vi "Day 3-1.vi"() -> ()   [LabVIEW 2022 SP3]
uses:
  <vilib>/Utility/miscctls.llb/LVMapReplaceAction.ctl
panel:
  out "sum 2":i32
  out "sum":i32
  in  "String":string="..172..............................454..46.......507..........809......923.778..................793..............137.............238........\n............*.........712........=.......*................515.*...........*.......690.........../..........658.........=.........*..........\n.........823.835........%.........710.....749........134..%............................#812...&.....925.../..........276.......386..........\n519..................13......341.................481....=.....$............-.......211.......92.......*.....................................\n............832*105..@........$..................*.........797.....535..932.........*....152...........123.........678.540...........-...6..\n....&..948..........................271....-....228..79.26.........................733...=...715............27.586........*.......883...*...\n..172.......=..+.............88&....%....340.55.....+.............465..398......=..................585.......*....*812...347................\n...........374.462.......166..................*...........786........*....*910..675.................*.....149................653*....+80....\n.......*............680.....*......876.........864..................259.................124.169....799............608..*.........98......951\n....615.......*....%.....151.........*....#802........$.......680......................../...............857........-.901...............*...\n..............3.................637..493...........926....636..*.....350........881.........699......886.../.458...........#..474*409...246.\n...&...336......922............*..........370..............$..581....*.....335.*.......608$..*..11.......$....-..........928................\n...50..*.........*...........978...453.....*.......-..22..........298.......*...711.........794...*...267............44*.......460....*.....\n...................................*........534..797....-.............61....272.....@874..........892.....707.............230....*..72.537..\n....................405............309..........................221./..*....................872%.......75..*......237.....*.................\n..208.176..239.........*172.............795.............670.......*..9..504......*.717..641........908*....975.....*......130...............\n.....*....*.......711$....................*..54.....494..../.333.882...........282....@.......927*....../.......555..983*...........479.....\n.915......670.524................866...862..@.........*../....*...................................72.901..................995..........&....\n...*..%.......*.....71.............*..................33.350.796.....612.............#..463..............*399.....=.......*......309........\n....8..951.886......@......41*......606.680...787................605*.....892.......219.*........972..846.........377....644................\n..............................718........*.......*.......355*688............*.145...................*.......576.............................\n..........867.*.....................+...974...148..........................87.#........500&...534..986..269...*.....576....302....+.........\n........@......504.......-........652.........................104....@502......................*...............691.*.........*.423..706..402\n.286..218.882........-....579......................320.....=...-..........48.393.....202......758.....242..951..............................\n....*.....*.....$..943.............928.....*......*......310......&........*....*...*......=..............*......295*133....................\n..698...331...859.......91.........#....815....822..............39..........833....749...591...........455....*..........&30....*...........\n............*............+..............................117............................%........727........256.439...19.......478...........\n......67.595...599.........442...997..187.................@.596..276..141.597*792...780.........*......*.............@..............#.......\n266@.............-..713.....*....*.......=..783...564*.......*.......@.........................839......255.............636......749..%.....\n........+............*.....963.926.39../......&.......274...228..../.....812.........487@.24.............................*..*..........348..\n...618...364.936.....708...........*....63..&.......................212....-..191..............798................*....591..906.............\n......./.....@...............591...127.......491...141..*.....+...............*......339.@483........204*......871.465..................%...\n....890..................997*............723........$..675..465..............372.875*.........%..........534.............209.......*.....648\n..............+................139*..........273..................../7.....-..............854.920...968%..........384......%.......830......\n......+632...273.......132*........793.........................207..........952..../..66..*........................#...........@............\n.......................................162..................35.*.................22..*....234..........468...................#.750..........\n.....15...161.....................93....@...818..-580........*.449...................125...........129....*................723......365.....\n.....-....*.......678.........&21...=....../..............547.......$.........701....................#.....845.........................#....\n743........634...*.................................................679...........*176......979....................928.......$..848..........\n...............107....296....845.....*..........@...........................69..............$..442.........960/...........311.*.............\n.........................*............519.....58..............248.......582*........403.......*........929..............-......486.......151\n....-390....396.........279.......718............449.....794..#..............+......*......251...980....../.../...328..476..................\n.............*.....................-......../...*...........*...292.........188...&..112............*315.....529............................\n713..........860......114.743&.......368.776...195.........850.=................943............543...................483*625................\n......889........=.../.................*.............916.............201............-...............426&....627..............284............\n.452...........579...........786.961.15.......488.......*373.....830*......947.645.189........367.................$..../551.................\n....*.....99*........388.793...*...*....578..../...........................*...%.......-497.........@221..720...885.........588....692......\n....................*........903..81.......*.......*........=./....615.....202...355........997-..........*................$.........*......\n...........780.@....259.439.................483....596...490..415....*............-........................683........*371...&644..964......\n.......796......161.......*..#884....................................458.247.500........145.895.62.742.267..........16......................\n......+............../.998...........173..511............552*847...%.....&.........+651..*.....*........*.....108........+..............*975\n.444.....560.297...149..............*....*......*...................173...................365............986.$............271...182...26....\n....*84....*......................#..471.696.736.107....974...-614............................../...%930..........................+......364\n............800...-155..235......446...................*....................286.......822../...199............670-....................%.....\n....882.................*.................521....*20.282.............641.......*..703*.....887......513*271....................+819..100....\n.99..*........933*...649.......407............922...............-......*....681.............................*....#426...204.................\n.....112................../.....*...819.94......................689...652...........182.933.858.............711...............610.....*437..\n.540..........#.........740...500....*...$....184.......................................*....#.......386...........................668......\n....$..........719..695...........824............&...882...........@......811........771.........142*.........867.667.*299.....143..........\n425....120.............*....401........................*....75..2..551.....*...719....................44..141...+..............+............\n...%..*..........963....209..&.....913.................871..=............%.904.........365.244.495....*....*........19......................\n.....971.........=.............883*.........225.967.............#......44.................*.....*..182......830.....@..190............487...\n...................................../........*.%........93....577..%......541.....*456.....370.52......................%.............@.....\n..82......396....................927..887...268...........&..........517...................%...............753................+.............\n.........*..........................*.........................................607..493.479.........521......*.....680*58..&....879..........\n......951.................136.&....585.........69....933.........25......265......*............923...&......5.............624........109....\n...........826..............$..407..............*...............*...+...........772.=...........*.............................628...........\n.......293..*...420...................................140.......728..815.196.-.......470.....403.................807..........*...99.....443\n......-.....732...*.........795....35........18.........*................*....789................931................-.52....727....*....*...\n.................477..@682..*.......*...118.........539.................844......................*...481.....%..........*..........863...773\n...479&......................585..817...@...........*...16*244...826*..........427...............694.......834.......949....................\n....................336....................-.....205..............................&............................................899..........\n....49...971...............331..289.......661.........400...57...-...................711......./873.........-...668...94......*.....42......\n.../.......#...........68...&...#...557.*.....425.......*...-..267.+.................*......#........@....993..=.......-....49......../.65..\n.............647..569.....*...........@..1...*......+...823.........579.............153...65...263....320..........243...........626........\n.......128...+.......*..215...%..684.........519..247.....................+.....................*...........320...*.................*.......\n........*..........827.......954...*.....378..........553..............434..........644....................*.......208............88..387...\n.907..402..............-..........16....*....%.........*...507..403.........*.................272...496....750.12.......................*...\n.............555.610.454.............322....954..529..25...*.....*../....651.43...534...........*......+.......$.........=...-121.442..709..\n.269*410......*...................................+.......163.608...451.........................999.....................292.................\n...........867....595*88.....#990...473.................................406.285.825......464...............378-..835&........%.......570*484\n.....550.............................-......162....812*37..................*.....*......+.................................693....%..........\n........*385...............*934..810.......*...................758..313........413..+.......265.691...559............807@.......824.608.....\n....373..................................580.....506..........*............852.......786....*.....*......*.........&...................*....\n.......%...932....194*688...713..................&.....333..410..817.524.....*...438.......410.129......312.....452......202..........146...\n.........=....+..............*....................................#..........626.*.....745.........974.....................+................\n580...212........485.........511.....495.768.361.....323-..............*176......595......*........*.......+.......147.........227....491...\n...*........%....*........85........*......*..*.............@..329$.623........*.......=..161.%...680...104.........$..452....*.........=...\n854..*489....33...992.......*......15...418..890...%......362............603.224.....431......701.............929.=....../.....408..........\n............................980..................428......................*......615..............%343............827..............686-.....\n48.213..................353.....%902......616.........583..%674.....361....711.........821&...31%.............................285...........\n...&...614.....@52.207#....*228............*..........*.............*..............................624.............734..........%.411*876...\n......*............................358...807.....280..174...232..715...$..............804..522........=........717..*..=....................\n434....262.655.822.358.&709...........*..........*..........=.........876.....952.............*................$...81.412.160....751........\n..................*.................976.......739..490*913.....@...........+....#.374..625..236..539........$...............................\n..743...................737@.............766....................197........878.....*....*...........*...861..32...............16...975......\n................972..@.....................&...293..85/.....561.......919..........156.............435....*..........835........*3..........\n........823.690.*....747...............799....*..........=....*........&...................241.........558...............459................\n....552*.....*...701.........................579.......187...691...#.*......694*980...........*.#...........244.............*....842........\n.57.......687.....................110*873........................469.217....................573..324.308*......%...........855....*..553....\n......551..................................................................142.......771*................902...................606..........\n.....*....990........869........8.......#477............330-....................37*......408.-751......-......239..........362..............\n...994...*..............=.984..*...194...............................972*967.......150...............433..517...*...........*........947....\n.........189..501*334...........56...#...............531...846...562..........477...............................19........396...570.*.......\n......................761..............243.....692......*.....*.....*.#985.......*...991-......=.320/.................%...........*.585.....\n....590.....&....$...$....993.554.....*.........%....132...623....429........549..31........643...................134.237........50.........\n.............385.538.....*....*.....826...........@....................................644......151*919......733.............73.....848.....\n.477...871..............5....68.841......80*.......405.70*898..............+25............*787..........368...*................/.......*....\n...*....*.....6....................*..=.....370......................................186.........146.......*...447.......287............611.\n443...893.....$.......%20.......108...43..........637......396...596............64......#.505...*.........141..............*......543.......\n.................197......244.................530.=...334.......*....335..745...../.......*......99..182..............645.963...............\n...........%....*........*.......593..704&..............-...@...211.....*......./.......571..178...............#.................+476.......\n.....*812..17.617.......249..327..-........527..15........238............926.564..............................260...........715*......../793\n....................826.........*............*.......................................@.........685.....@................954.....423.........\n.............796*..............260..946.....848...902.............285......136....211............*.....258.874.....332.*....................\n....&829.........348....539.........*............*....623....*.....&.........*..........252.%253..86......../..599.*...592.......672-.232...\n............752.........-.........375............859....*.926.182....733......241......=..............276..........762................*.....\n.............................482...........346........374...........&............................493.....*322..........................175..\n...*../........793..&532.........530..........*...........509.861.......134........353............*....................*94..................\n480....761........+.....................=..768..790..@......&.*....296.................311........340...344.....989.142..........411........\n.............208.......300.............506......*.....267.....918....*.......204..........%.606.........*....+...=.......*397.......*...257.\n............+.........*......-...............636..476................109......*.............*......-....115...91......823........929....@...\n...595........313.....849.452......568...............%..802....................915...730....138.30..455.....................589.............\n..............*................290....%.......147..........#....492..83....12*........=.........*.............................@.......17....\n970.....+.-...701....#264....%....$.......113.......916........*..............620............809........$788....@.....446........904..*.....\n...*..221.112..............610............@.....799............713........657.......325..........................551..*.............=..615..\n.295...............852..........*....986.........*..........................................-............620..........665.....930...........\n.....785.......542.*............732...=........583...+....................424....$....702.367..993.......*....386..#.............*..........\n........*...........114....704..........377...........633...........=730...#..241.......%.....*.....-.396...........372......135..806.......\n.......122......963........$............*.....................509$........................50.....280.........672.........538..$........619..\n.....................957.....542...731..941.......*....59..........571*554....214....108.@...............104*............=.............*....\n.....=...............*.......*....../.............337./...........................=..%..........................................873..563....\n....771..500........868.......213......902....456........../.........255.....377.781......=348................133..@...367*696.....*........\n........*....$..25........784..................$...........735..413.....*108./............................645...*..8............185.........\n..603.389..956.*...........*.......636...866.....338...+25......*...+..........................................667........#..........+..296.\n...*............544.....510..418.=....=....*....................379.478.....961.............410&...........413......*912..469..758.733..-...\n798....*565.793.............*....98.....447.....@......291...$...............*..244................%..491.../...................*...........\n....546......*....454...120..683.............923.....@...*...865.574......276........56......57.659..*................-...-...512...........\n............329...*.................................606.599...................*927..*.........-.......674..*........723..974................\n................378..911........987.....606......................899.73....489......848.....................664...............388......589.."
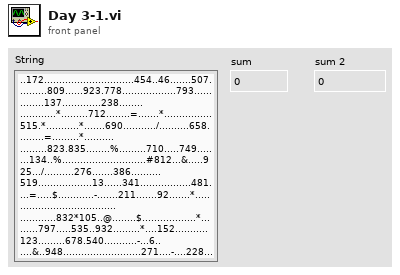
[diagram p1: front panel]
types:
  T1 = cluster{"Symbol":string, "Start":cluster{"Row":i32, "Col":i32}, "End":cluster{"Row":i32, "Col":i32}}
  T2 = cluster{"Number":i32, "Start":cluster{"Row":i32, "Col":i32}, "End":cluster{"Row":i32, "Col":i32}}
  T3 = cluster{i32, cluster{i32, i32}, cluster{i32, i32}, cluster{"String":string, cluster{i32, i32}}[]}
  T4 = typedef "LVMapReplaceAction.ctl" = enum32{"Modify Entry only if found", "Add or Modify Entry", "Delete Entry"}
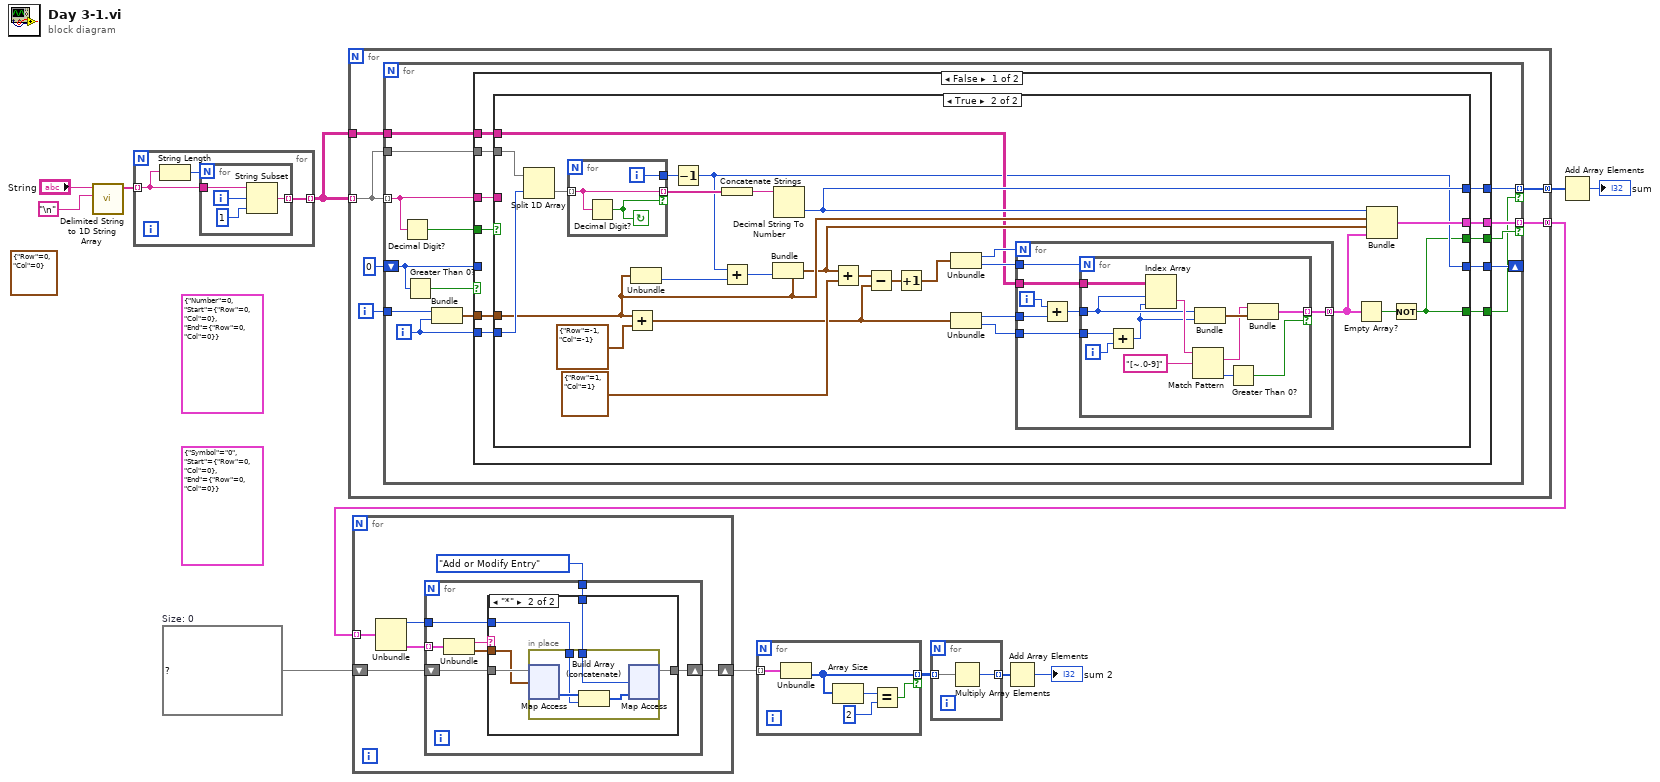
[diagram p0: block diagram]
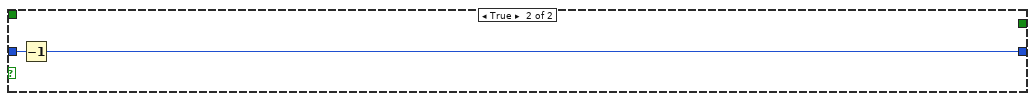
[diagram p4: hidden frame]
diagram:
  w5 = map{cluster{"Row":i32, "Col":i32}, i32[]} {}  # Size: 0
  (unwired) T1 {"Symbol"="0", "Start"={"Row"=0, "Col"=0}, "End"={"Row"=0, "Col"=0}}
  (unwired) T2 {"Number"=0, "Start"={"Row"=0, "Col"=0}, "End"={"Row"=0, "Col"=0}}
  (unwired) cluster{"Row":i32, "Col":i32} {"Row"=0, "Col"=0}
  n1 = call <vilib>:"Delimited String to 1D String Array.vi"("delimiter"="\n", "delimited string"="String") -> ("string array"=w10:string[])  [unwired: 9 in]
  n2 = for {
    tunnel: w10 -> [w14] mode=indexing
    tunnel: [w13] -> w7 mode=indexing
    n3 = String Length(string=w14) -> (length=w15:i32)
    n4 = for {
      N: w15 -> [_]
      tunnel: w14 -> [w19]
      tunnel: [w16] -> w13 mode=indexing
      i -> [w18]
      n5 = String Subset(string=w19, offset (0)=w18, length (rest)=1 ("length (rest)")) -> (substring=w16:string)
    }
  }
  n6 = for {
    tunnel: w7 -> [w23] mode=indexing
    tunnel: [w22] -> w6 mode=concatenating
    tunnel: [w21] -> w9 mode=concatenating
    tunnel: w7 -> [w20]
    i -> [w24]
    n7 = for {
      tunnel: w23 -> [w35] mode=indexing
      shift-right: [w37] -> _
      shift-left: 0 -> [w38]
      tunnel: w24 -> [w34]
      tunnel: w23 -> [w32]
      tunnel: [w30] -> w22 mode=indexing if=w28
      tunnel: [w29] -> w21 mode=indexing if=w26
      tunnel: w20 -> [w27]
      i -> [w31]
      n8 = Decimal Digit?(1:w35) -> (0:w36:bool)
      n9 = Greater Than 0?(x=w38) -> (x > 0?=w39:bool)
      n10 = Bundle(w34, w31) -> (w33:cluster{i32, i32})  [unwired: 1 in]
      n11 = case shown="False" w39 {
        tunnel: w38 -> [_ w101]
        tunnel: [w45 w100] -> w37
        tunnel: w36 -> [w50 _]
        tunnel: w35 -> [w49 _]
        tunnel: w33 -> [w48 _]
        tunnel: w32 -> [w47 _]
        tunnel: w31 -> [w46 _]
        tunnel: [w44 _] -> w30
        tunnel: [w43 _] -> w28
        tunnel: [w42 _] -> w29
        tunnel: w27 -> [w41 _]
        tunnel: [w40 _] -> w26
        frame False {
          n12 = case shown="True" w50 {
            tunnel: w49 -> [_ _]
            tunnel: w48 -> [_ w67]
            tunnel: w47 -> [_ w77]
            tunnel: w46 -> [_ w76]
            tunnel: [_ w53] -> w45
            tunnel: [_ w69] -> w44
            tunnel: [_ w51] -> w43
            tunnel: [_ w68] -> w42
            tunnel: w41 -> [_ w59]
            tunnel: [_ w51] -> w40
            frame False {
            }
            frame True {
              n13 = Split 1D Array(array=w77, index=w76) -> (second subarray=w75:string[])  [unwired: 1 out]
              n14 = for {
                tunnel: w75 -> [w99] mode=indexing
                tunnel: [w99] -> w74 mode=indexing if=w98
                tunnel: [w97] -> w71
                i -> [w97]
                stop <- w98 continue-if-true
                n15 = Decimal Digit?(1:w99) -> (0:w98:bool)
              }
              n16 = Add(x=w67, y=cluster{"Row":i32, "Col":i32} {"Row"=-1, "Col"=-1}) -> (x+y=w58:cluster{i32, i32})
              n17 = Unbundle(w67) -> (w72:i32)  [unwired: 1 out]
              n18 = Decrement(x=w71) -> (x-1=w53:i32)
              n19 = Concatenate Strings(w74) -> (w73:string)
              n20 = Add(x=w53, y=w72) -> (x+y=w70:i32)
              n21 = Bundle(cluster=w67, w70) -> (w65:cluster{i32, i32})  [unwired: 1 in]
              n22 = Decimal String To Number(string=w73) -> (number=w68:i32)  [unwired: 2 in, 1 out]
              n23 = Add(x=w65, y=cluster{"Row":i32, "Col":i32} {"Row"=1, "Col"=1}) -> (x+y=w63:cluster{i32, i32})
              n24 = Subtract(x=w63, y=w58) -> (x-y=w62:cluster{i32, i32})
              n25 = Increment(x=w62) -> (x+1=w52:cluster{i32, i32})
              n26 = Unbundle(w52) -> (w61:i32, w60:i32)
              n27 = Unbundle(w58) -> (w57:i32, w56:i32)
              n28 = for {
                N: w61 -> [_]
                tunnel: w60 -> [w84]
                tunnel: w59 -> [w83]
                tunnel: w57 -> [w82]
                tunnel: w56 -> [w79]
                tunnel: [w78] -> w55 mode=concatenating
                i -> [w81]
                n29 = Add(x=w81, y=w82) -> (x+y=w80:i32)
                n30 = for {
                  N: w84 -> [_]
                  tunnel: w83 -> [w94]
                  tunnel: w80 -> [w91]
                  tunnel: w79 -> [w96]
                  tunnel: [w86] -> w78 mode=indexing if=w85
                  i -> [w95]
                  n31 = Add(x=w96, y=w95) -> (x+y=w90:i32)
                  n32 = Index Array(array=w94, index (row)=w91, index (col)=w90) -> (element=w93:string)
                  n33 = Match Pattern(string=w93, regular expression="[~.0-9]") -> (match substring=w88:string, offset past match=w87:i32)  [unwired: 1 in, 2 out]
                  n34 = Bundle(w91, w90) -> (w89:cluster{i32, i32})  [unwired: 1 in]
                  n35 = Greater Than 0?(x=w87) -> (x > 0?=w85:bool)
                  n36 = Bundle("String"=w88, w89) -> (w86:cluster{"String":string, cluster{i32, i32}})  [unwired: 1 in]
                }
              }
              n37 = Empty Array?(array=w55) -> (empty?=w54:bool)
              n38 = Bundle(w68, w67, w65, w55) -> (w69:T3)  [unwired: 1 in]
              n39 = Not(x=w54) -> (.not. x?=w51:bool)
            }
          }
        }
        frame True {
          n40 = Decrement(x=w101) -> (x-1=w100:i32)
        }
      }
    }
  }
  n41 = for {
    tunnel: w6 -> [w107] mode=indexing
    shift-right: [w102] -> w4
    shift-left: w5 -> [w104]
    n42 = Unbundle(w107) -> (w105:i32, w106:cluster{"String":string, cluster{i32, i32}}[])  [unwired: 2 out]
    n43 = for {
      tunnel: w106 -> [w114] mode=indexing
      tunnel: w105 -> [w112]
      shift-right: [w110] -> w102
      shift-left: w104 -> [w111]
      tunnel: LVMapReplaceAction."Add or Modify Entry" ("action") -> [w108]
      n44 = Unbundle(w114) -> ("String"=w113:string, w109:cluster{i32, i32})
      n45 = case shown="\"*\"" w113 {
        tunnel: w112 -> [_ w117]
        tunnel: w111 -> [w115 w120]
        tunnel: [w115 w116] -> w110
        tunnel: w109 -> [_ w119]
        tunnel: w108 -> [_ w118]
        frame Default {
        }
        frame "*" {
          n46 = in-place {
            in-place-border: w118 -> [w124]
            in-place-border: w117 -> [w122]
            n47 = in-place-map #1(w120, w119) -> (w123:i32[])  [unwired: 1 in, 1 out]
            n48 = Build Array (concatenate)(w123, w122) -> (w121:i32[])
            n49 = in-place-map #1(w121, w124) -> (w116:map{cluster{"Row":i32, "Col":i32}, i32[]})  [unwired: 2 out]
          }
        }
      }
    }
  }
  n50 = for {
    tunnel: w4 -> [w129] mode=indexing
    tunnel: [w126] -> w3 mode=indexing if=w125
    n51 = Unbundle(w129) -> (w126:i32[])  [unwired: 1 out]
    n52 = Array Size(array=w126) -> (size(s)=w128:i32)
    n53 = Equal?(x=w128, y=2) -> (x = y?=w125:bool)
  }
  n54 = for {
    tunnel: w3 -> [w131] mode=indexing
    tunnel: [w130] -> w2 mode=indexing
    n55 = Multiply Array Elements(1:w131) -> (0:w130:i32)
  }
  n56 = Add Array Elements(numeric array=w2) -> (sum=→"sum 2":i32)
  n57 = Add Array Elements(numeric array=w9) -> (sum=→"sum":i32)
